vi "LV_UDP_client.vi"() -> ()   [LabVIEW 2020]
panel:
  in  "Send Image":bool
  out "Path to Python script":path
  out "error out":errorcluster
  in  "Stop":bool
  out "Answer":string
  in  "Ping":bool
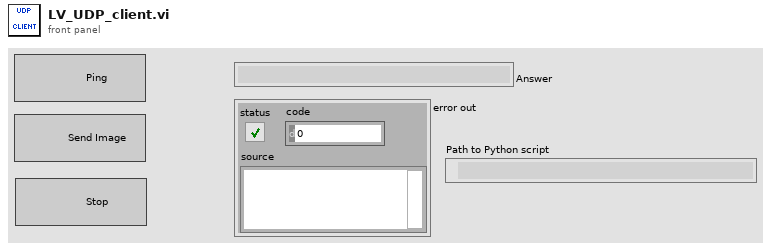
[diagram p1: front panel]
types:
  T1 = enum8{"Enabled", "Disabled", "Disabled and Grayed Out"}
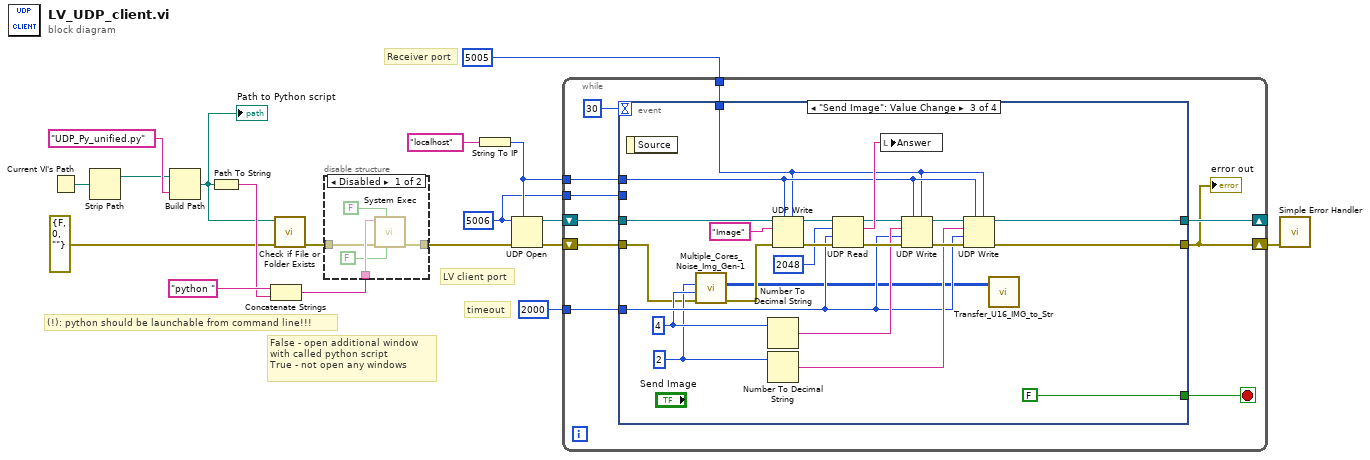
[diagram p0: block diagram]
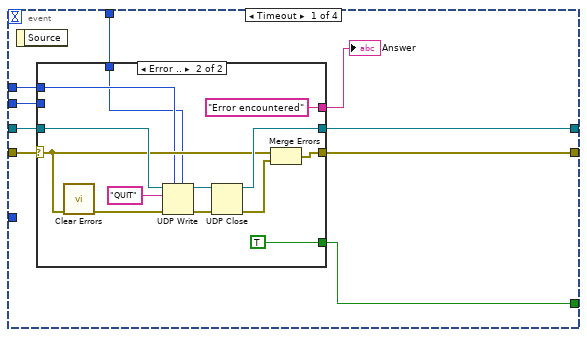
[diagram p3: hidden frame]
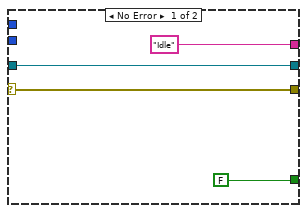
[diagram p4: hidden frame]
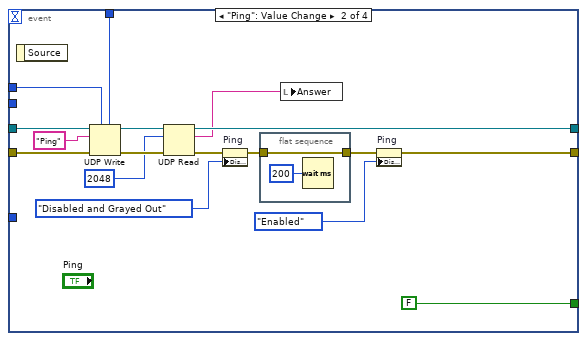
[diagram p5: hidden frame]
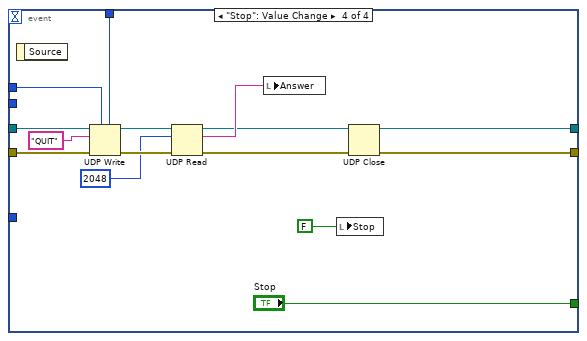
[diagram p6: hidden frame]
diagram:
  w3 = u16 5006 ("remote port or service name")
  # "timeout"
  # "Receiver port"
  # "LV client port"
  # "False - open additional window\nwith called python script\nTrue - not open any windows"
  # "(!): python should be launchable from command line!!!"
  n1 = Current VI's Path() -> (path=w17:path)
  n2 = Strip Path(path=w17) -> (stripped path=w12:path)  [unwired: 1 out]
  n3 = Build Path(base path=w12, name or relative path="UDP_Py_unified.py" ("string")) -> (appended path=w10:path)
  "Path to Python script" <- w10
  n4 = Path To String(path=w10) -> (string=w13:string)
  n5 = Concatenate Strings("python " ("command line"), w13) -> (w15:string)
  n6 = call <vilib>:"Check if File or Folder Exists.vi"("error in (no error)"=errorcluster {"status"=FALSE, "code"=0, "source"=""}, "path"=w10) -> ("error out"=w9:errorcluster)  [unwired: 7 in, 2 out]
  n7 = disable-structure shown="Disabled" {
    disable-tunnel: w15 -> [w23 _]
    disable-tunnel: [w22 w24] -> w8
    disable-tunnel: w9 -> [w20 w24]
    frame Disabled {
      n8 = call <vilib>:"System Exec.vi"("run minimized? (F)"=FALSE, "wait until completion? (T)"=FALSE, "error in (no error)"=w20, "command line"=w23) -> ("error out"=w22:errorcluster)  [unwired: 4 in, 3 out]
    }
    frame Enabled {
    }
  }
  n9 = String To IP(1:"localhost" ("address")) -> (0:w4:u32)
  n10 = UDP Open(7:w4, 8:w8, 11:w3) -> (port=w6:refnum<k16>, 0:w7:errorcluster)  [unwired: 2 in, 1 out]
  n11 = while {
    shift-right: [w31] -> _
    shift-left: w6 -> [w32]
    shift-right: [w29] -> w18
    shift-left: w7 -> [w33]
    tunnel: w4 -> [w27]
    tunnel: w3 -> [w28]
    tunnel: u16 5005 ("remote port or service name") -> [w26]
    tunnel: 2000 -> [w25]
    stop <- w30 stop-if-true
    n12 = event shown="[2] \"Send Image\": Value Change" {
      selector: _ -> [_ _ _ _]
      dyn-events: _ -> [_ _ _ _]
      timeout: 30 -> [_ _ _ _]
      tunnel: [w39 FALSE ("Stop") FALSE ("Stop") "Stop"] -> w30
      tunnel: w33 -> [w43 w71 w82 w112]
      tunnel: w32 -> [w42 w70 w101 w113]
      tunnel: [w41 w66 w88 w114] -> w31
      tunnel: [w40 w73 w90 w115] -> w29
      tunnel: w28 -> [w37 _ _ _]
      tunnel: w27 -> [w36 w62 w92 w104]
      tunnel: w26 -> [w35 w61 w91 w103]
      tunnel: w25 -> [_ _ w85 _]
      event Timeout {
        n13 = event-data() -> ()  [unwired: 1 in, 1 out]
        n14 = case shown="Error .." w43 {
          selector: w43 -> [w46 w51]
          tunnel: [w47 w58] -> w41
          tunnel: w42 -> [w47 w57]
          tunnel: [w46 w52] -> w40
          tunnel: [FALSE ("Stop") TRUE ("Stop")] -> w39
          tunnel: ["Idle" ("Answer") "Error encountered" ("Answer")] -> w38
          tunnel: w37 -> [_ _]
          tunnel: w36 -> [_ w49]
          tunnel: w35 -> [_ w48]
          frame No Error {
          }
          frame Error {
            n15 = call <vilib>:"Clear Errors.vi"("error in (no error)"=w51) -> ("error out"=w56:errorcluster)  [unwired: 5 in, 1 out]
            n16 = UDP Write(address=w49, port or service name=w48, connection ID=w57, data in="QUIT", 8:w56) -> (error out=w55:errorcluster, 3:w53:refnum<k16>)  [unwired: 1 in]
            n17 = UDP Close(connection ID=w53, 8:w55) -> (connection ID out=w58:refnum<k16>, error out=w50:errorcluster)
            n18 = Merge Errors(w51, w50) -> (w52:errorcluster)
          }
        }
        "Answer" <- w38
      }
      event "Ping": Value Change {
        n19 = event-data() -> ()  [unwired: 1 in, 1 out]
        n20 = UDP Write(address=w62, port or service name=w61, connection ID=w70, data in="Ping", 8:w71) -> (error out=w68:errorcluster, 3:w67:refnum<k16>)  [unwired: 1 in]
        n21 = UDP Read(connection ID=w67, max size (548)=2048 ("bytes to read"), 8:w68) -> (data out=w63:string, error out=w65:errorcluster, 3:w66:refnum<k16>)  [unwired: 1 in, 2 out]
        n22 = property on="Ping" class="Bool"(error in=w65, "DisabledEnum"=T1."Disabled and Grayed Out" ("Disabled")) -> (error out=w76:errorcluster)  [unwired: 1 in, 1 out]
        n23 = flat-sequence {
          tunnel: w76 -> [w78]
          tunnel: [w78] -> w74
          frame #0 {
            n24 = Wait (ms)(milliseconds to wait=u32 200) -> ()  [unwired: 1 out]
          }
        }
        n25 = local write "Answer"(w63) -> ()
        n26 = property on="Ping" class="Bool"(error in=w74, "DisabledEnum"=T1."Enabled" ("Disabled")) -> (error out=w73:errorcluster)  [unwired: 1 in, 1 out]
      }
      event "Send Image": Value Change {
        w83 = 2 ("number")
        w84 = 4 ("number")
        n27 = event-data() -> ()  [unwired: 1 in, 1 out]
        n28 = call "Multiple_Cores_Noise_Img_Gen-1.vi"("error IN"=w82, "[IN] Width"=w84, "[IN] Height"=w83) -> ("error OUT"=w81:errorcluster, "[OUT] U16 Pixel Img"=w80:u16[][])  [unwired: 7 in]
        n29 = Number To Decimal String(number=w84) -> (decimal integer string=w87:string)  [unwired: 1 in]
        n30 = Number To Decimal String(number=w83) -> (decimal integer string=w86:string)  [unwired: 1 in]
        n31 = UDP Write(address=w92, port or service name=w91, connection ID=w101, data in="Image", 8:w81) -> (error out=w100:errorcluster, 3:w99:refnum<k16>)  [unwired: 1 in]
        n32 = UDP Read(connection ID=w99, max size (548)=2048 ("bytes to read"), timeout ms (25000)=w85, 8:w100) -> (data out=w97:string, error out=w95:errorcluster, 3:w96:refnum<k16>)  [unwired: 2 out]
        n33 = local write "Answer"(w97) -> ()
        n34 = UDP Write(address=w92, port or service name=w91, connection ID=w96, data in=w87, 8:w95, 9:w85) -> (error out=w94:errorcluster, 3:w93:refnum<k16>)
        n35 = UDP Write(address=w92, port or service name=w91, connection ID=w93, data in=w86, 8:w94, 9:w85) -> (error out=w90:errorcluster, 3:w88:refnum<k16>)
        n36 = call "Transfer_U16_IMG_to_Str.vi"("[IN] U16 Pixel Img"=w80) -> ()  [unwired: 2 in, 1 out]
      }
      event "Stop": Value Change {
        n37 = event-data() -> ()  [unwired: 1 in, 1 out]
        n38 = UDP Write(address=w104, port or service name=w103, connection ID=w113, data in="QUIT", 8:w112) -> (error out=w109:errorcluster, 3:w110:refnum<k16>)  [unwired: 1 in]
        n39 = UDP Read(connection ID=w110, max size (548)=2048 ("bytes to read"), 8:w109) -> (data out=w107:string, error out=w108:errorcluster, 3:w106:refnum<k16>)  [unwired: 1 in, 2 out]
        n40 = local write "Answer"(w107) -> ()
        n41 = local write "Stop"(FALSE ("Stop")) -> ()
        n42 = UDP Close(connection ID=w106, 8:w108) -> (connection ID out=w114:refnum<k16>, error out=w115:errorcluster)
      }
    }
    "error out" <- w29
  }
  n43 = call <vilib>:"Simple Error Handler.vi"("error in (no error)"=w18) -> ()  [unwired: 4 in, 5 out]
